vi "killambient.vi"() -> ()   [LabVIEW 2011]
panel:
  in  "text":string="kill"
  in  "path":path=path "/tmp/atlas/ambientpipe"
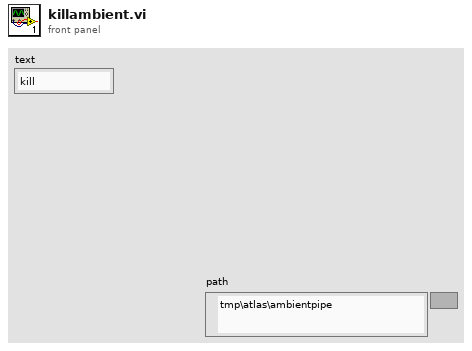
[diagram p1: front panel]
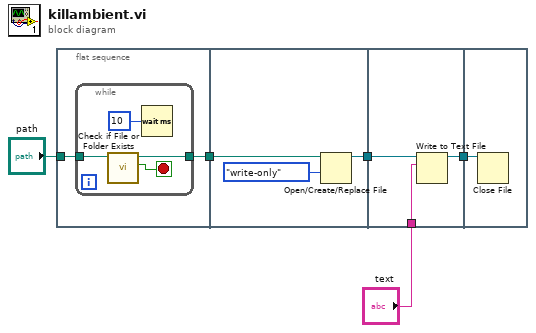
[diagram p0: block diagram]
diagram:
  n1 = flat-sequence {
    tunnel: "path" -> [w7]
    tunnel: [w6] -> w4
    tunnel: w4 -> [w14]
    tunnel: [w12] -> w3
    tunnel: w3 -> [w17]
    tunnel: [w16] -> w2
    tunnel: "text" -> [w15]
    tunnel: w2 -> [w18]
    frame #0 {
      n2 = while {
        tunnel: w7 -> [w9]
        tunnel: [w8] -> w6
        stop <- w10 stop-if-true
        n3 = call <vilib>:"Check if File or Folder Exists.vi"("path"=w9) -> ("file or folder exists?"=w10:bool, "dup path"=w8:path)  [unwired: 8 in, 1 out]
        n4 = Wait (ms)(milliseconds to wait=u32 10) -> ()  [unwired: 1 out]
      }
    }
    frame #1 {
      n5 = Open/Create/Replace File(file path (use dialog)=w14, access (0:read/write)=enum16{"read/write", "read-only", "write-only"}."write-only") -> (refnum out=w12:refnum<file>)  [unwired: 4 in, 2 out]
    }
    frame #2 {
      n6 = Write to Text File(file (use dialog)=w17, text=w15) -> (refnum out=w16:refnum<file>)  [unwired: 2 in, 2 out]
    }
    frame #3 {
      n7 = Close File(refnum=w18) -> ()  [unwired: 1 in, 2 out]
    }
  }
